vi "TirarBolaDaParede.vi"(8 "Parede":T6(ring), 9 "balls":T8[](array[typedef]), 10 "Robot in":T1, 11 "IA State":T7={"our_robots"=[], "enemy_robots"=[], "balls"=[], "geometry"={"field_length"=0, "field_width"=0, "goal_width"=0, "goal_depth"=0, "center_circle_radius"=0, "defense_width"=0, "defense_depth"=0, "free_kick_from_defense_dist"=0, "penalty_spot_from_field_line_dist"=0, "penalty_line_from_spot_dist"=0, "half_moon_depth"=0, "half_moon_width"=0}, "IA Judge"={"stage"="", "command"="", "our_goalie_id"=0.0, "enemy_goalie_id"=0.0, "command enum"=enum."Halt", "Time"=enum."Azul"}, "Received Timestamp"=timestamp(0 s since 1904-01-01), "Events"={"Touch"=FALSE, "id touch"=0.0, "Ball out of \nVision"=FALSE, "Ball inside \nGoalie area"=FALSE, "Robot not responding"=FALSE, "Robots responding status"=[1.0, 1.0, 1.0, 1.0, 1.0, 1.0], "Enemy Ball \nPossession"=FALSE, "Id ini Possession"=0.0, "Ball Possesion"=FALSE, "Id Possesion"=0.0, "Ball at\nour goal side"=FALSE, "Ball at\ntouchline"=FALSE, "Ball at\nenemy goal side"=FALSE}}) -> (3 "Cluster de saída":T1)   [LabVIEW 2018]
doc: "Função que lida com o atacante quando em \"Tirar a bola da parede\"."
uses:
  Core/AI Robot.ctl
  Intel/Functions Enum.ctl
  Intel/AttackerStates.ctl
  Path Planning/RRT/PathDests.ctl
  Path Planning/RRT/PathDest.ctl
  Core/AI Ball.ctl
  Core/AI Input.ctl
  Core/Field Size.ctl
  Core/AI Judge.ctl
  Intel/Command Enum.ctl
  Util/Events/Events.ctl
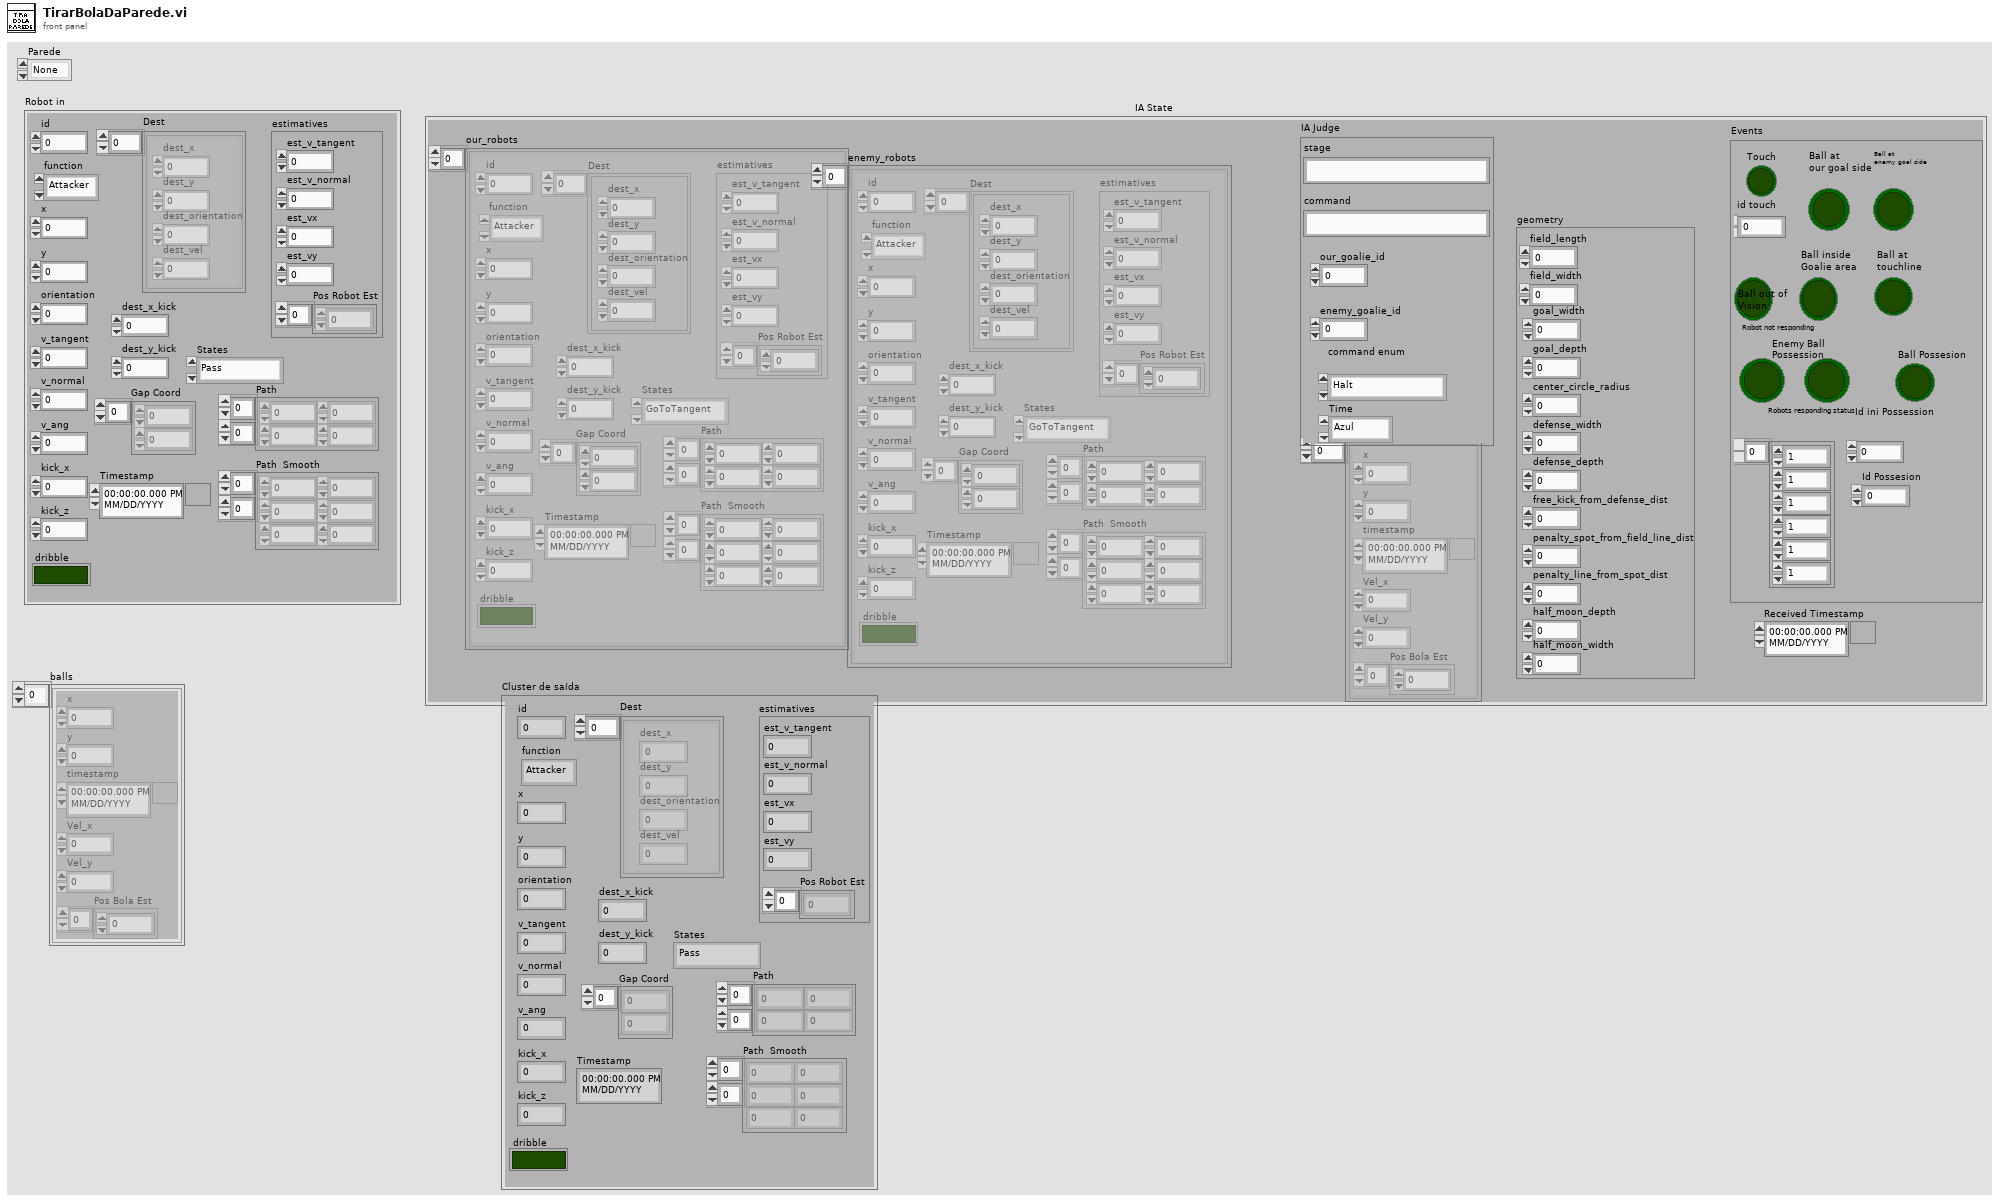
[diagram p1: front panel]
types:
  T1 = typedef "AI Robot.ctl" = cluster{"id":u32, "function":T2, "x":dbl, "y":dbl, "orientation":dbl, "v_tangent":dbl, "v_normal":dbl, "v_ang":dbl, "kick_x":dbl, "kick_z":dbl, "dribble":bool, "Timestamp":timestamp, "estimatives":cluster{"est_v_tangent":dbl, "est_v_normal":dbl, "est_vx":dbl, "est_vy":dbl, "Pos Robot Est":dbl[]}, "dest_x_kick":dbl, "dest_y_kick":dbl, "Gap Coord":dbl[], "States":T3, "Path ":dbl[][], "Path  Smooth":dbl[][], "Dest":T4}
  T2 = typedef "Functions Enum.ctl" = enum16{"Attacker", "Goalie", "Defender", "Striker", "Goto 0", "Dummy", "Kicker", "ZigZag"}
  T3 = typedef "AttackerStates.ctl" = enum16{"Pass", "GoToTangent", "BallGetting", "GoToKick", "Rotate anti-clockwise", "Rotate Clockwise", ""}
  T4 = typedef "PathDests.ctl" = T5[]
  T5 = typedef "PathDest.ctl" = cluster{"dest_x":dbl, "dest_y":dbl, "dest_orientation":dbl, "dest_vel":dbl}
  T6 = enum16{"None", "Frente", "Trás", "Cima", "Baixo"}
  T7 = typedef "AI Input.ctl" = cluster{"our_robots":T1[], "enemy_robots":T1[], "balls":T8[], "geometry":T9, "IA Judge":T10, "Received Timestamp":timestamp, "Events":T12}
  T8 = typedef "AI Ball.ctl" = cluster{"x":dbl, "y":dbl, "timestamp":timestamp, "Vel_x":dbl, "Vel_y":dbl, "Pos Bola Est":dbl[]}
  T9 = typedef "Field Size.ctl" = cluster{"field_length":u32, "field_width":u32, "goal_width":u32, "goal_depth":u32, "center_circle_radius":u32, "defense_width":u32, "defense_depth":u32, "free_kick_from_defense_dist":u32, "penalty_spot_from_field_line_dist":u32, "penalty_line_from_spot_dist":u32, "half_moon_depth":u32, "half_moon_width":u32}
  T10 = typedef "AI Judge.ctl" = cluster{"stage":string, "command":string, "our_goalie_id":dbl, "enemy_goalie_id":dbl, "command enum":T11, "Time":enum16{"Azul", "Amarelo"}}
  T11 = typedef "Command Enum.ctl" = enum16{"Halt", "Stop", "Force Start", "PKA Normal Start", "Prepare Kickoff Ally", "PKE Normal Start", "Prepare Kickoff Enemy", "Prepare Penalty Ally", "PPA Normal Start", "Prepare Penalty Enemy", "PPE Normal Start", "Ball Placement Enemy Up", "Ball Placement Enemy Down", "Ball Placement Ally Up", "Ball Placement Ally Mid", "Ball Placement Ally Down", "Indirect Free Enemy", "Indirect Free Ally", "Timeout Enemy", "Timeout Ally", "Goal Enemy", "Goal Ally", "Normal Half Time", "Extra Time Break", "Extra Half Time", "None", "Post Game"}
  T12 = typedef "Events.ctl" = cluster{"Touch":bool, "id touch":dbl, "Ball out of \nVision":bool, "Ball inside \nGoalie area":bool, "Robot not responding":bool, "Robots responding status":dbl[], "Enemy Ball \nPossession":bool, "Id ini Possession":dbl, "Ball Possesion":bool, "Id Possesion":dbl, "Ball at\nour goal side":bool, "Ball at\ntouchline":bool, "Ball at\nenemy goal side":bool}
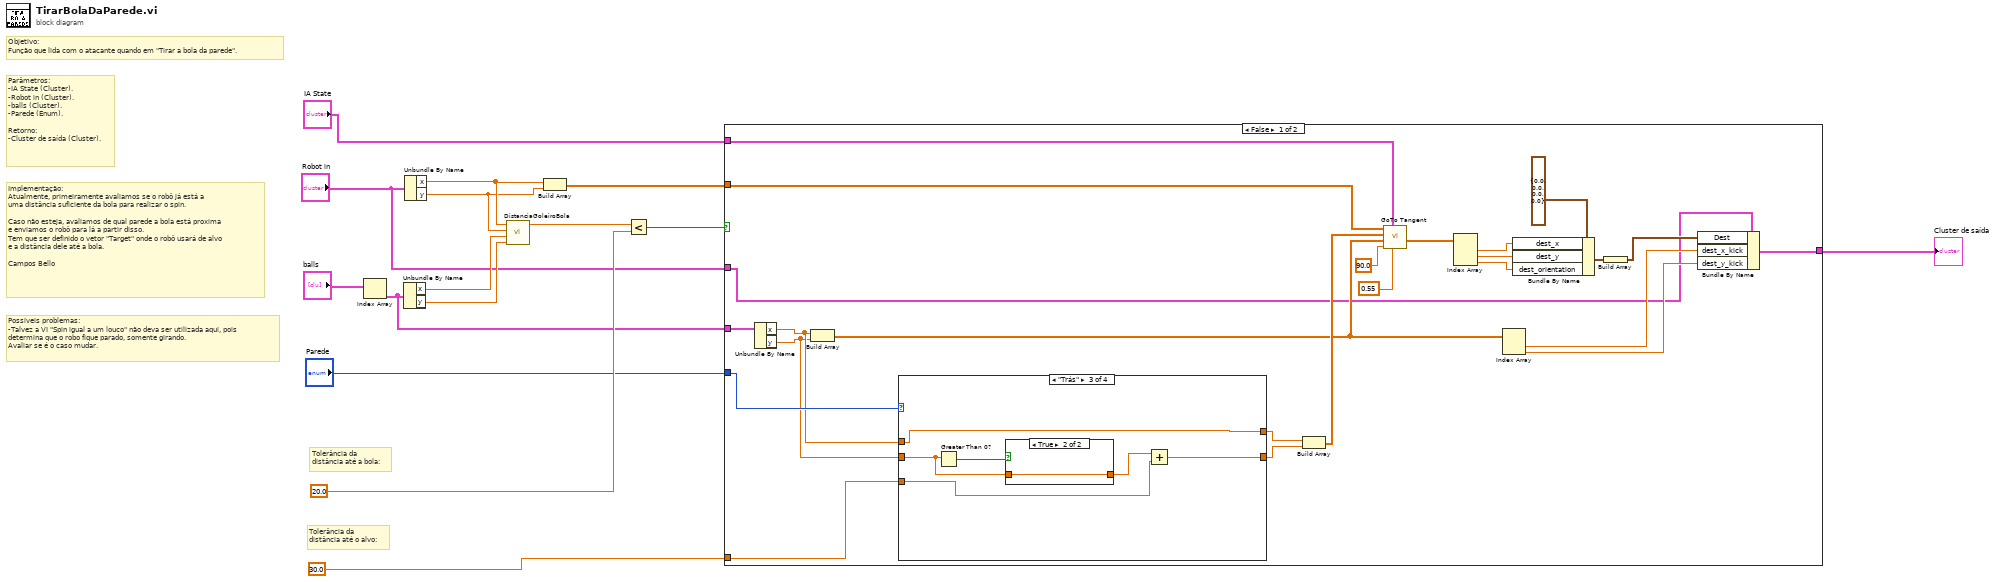
[diagram p0: block diagram]
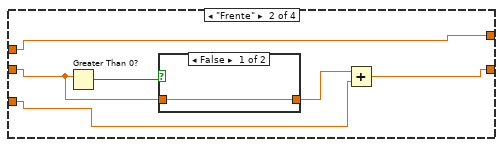
[diagram p3: hidden frame]
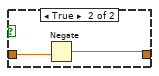
[diagram p4: hidden frame]
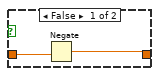
[diagram p5: hidden frame]
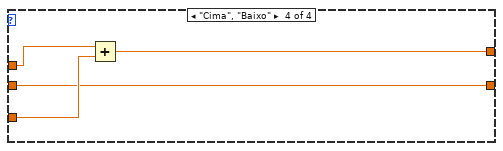
[diagram p6: hidden frame]
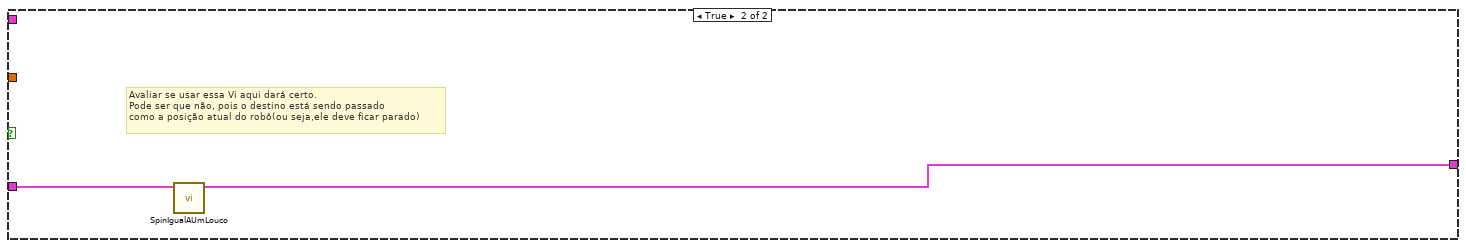
[diagram p7: hidden frame]
diagram:
  # "Possiveis problemas:\n-Talvez a VI \"Spin igual a um louco\" não deva ser utilizada aqui, pois\ndetermina que o robo fique parado, somente girando.\nAvaliar se é o caso mudar."
  # "Implementação:\nAtualmente, primeiramente avaliamos se o robô já está a\numa distância suficiente da bola para realizar o spin.\n\nCaso não esteja, avaliamos de qual parede a bola está proxima\ne enviamos o robô para lá a partir disso.\nTem que ser definido o vetor \"Target\" onde o robô usará de alvo\ne a distância dele até a bola.\n\nCampos Bello"
  # "Parâmetros:\n-IA State (Cluster).\n-Robot in (Cluster).\n-balls (Cluster).\n-Parede (Enum).\n\nRetorno:\n-Cluster de saída (Cluster)."
  # "Objetivo:\nFunção que lida com o atacante quando em \"Tirar a bola da parede\"."
  # "Tolerância da\ndistância até o alvo:"
  # "Tolerância da\ndistância até a bola:"
  n1 = Index Array(array="balls") -> (element=w8:T8)  [unwired: 1 in]
  n2 = Unbundle By Name(w8) -> ("x"=w14:dbl, "y"=w13:dbl)
  n3 = Unbundle By Name("Robot in") -> ("x"=w7:dbl, "y"=w6:dbl)
  n4 = call "DistanciaGoleiroBola.vi"("Y bola"=w13, "X bola"=w14, "Y goleiro"=w6, "X goleiro"=w7) -> ("Distância"=w12:dbl)  [unwired: 7 in]
  n5 = Build Array(w7, w6) -> (w5:dbl[])
  n6 = Less?(x=w12, y=20.0) -> (x < y?=w10:bool)
  n7 = case shown="False" w10 {
    tunnel: "Robot in" -> [w17 w65]
    tunnel: [w16 w64] -> w1
    tunnel: w8 -> [w39 _]
    tunnel: w5 -> [w38 _]
    tunnel: "IA State" -> [w37 _]
    tunnel: "Parede" -> [w34 _]
    tunnel: 30.0 -> [w31 _]
    frame False {
      n8 = Unbundle By Name(w39) -> ("x"=w33:dbl, "y"=w32:dbl)
      n9 = Build Array(w33, w32) -> (w21:dbl[])
      n10 = case shown="\"Trás\"" w34 {
        tunnel: w33 -> [w41 w44 w52 w63]
        tunnel: w32 -> [w40 w45 w55 w61]
        tunnel: w31 -> [_ w42 w53 w62]
        tunnel: [w40 w43 w51 w61] -> w29
        tunnel: [w41 w44 w52 w60] -> w30
        frame "None", Default {
        }
        frame "Frente" {
          n11 = Greater Than 0?(x=w45) -> (x > 0?=w47:bool)
          n12 = case shown="False" w47 {
            tunnel: w45 -> [w48 w50]
            tunnel: [w48 w49] -> w46
            frame False {
            }
            frame True {
              n13 = Negate(x=w50) -> (-x=w49:dbl)
            }
          }
          n14 = Add(x=w46, y=w42) -> (x+y=w43:dbl)
        }
        frame "Trás" {
          n15 = Greater Than 0?(x=w55) -> (x > 0?=w56:bool)
          n16 = case shown="True" w56 {
            tunnel: w55 -> [w58 w59]
            tunnel: [w57 w59] -> w54
            frame False {
              n17 = Negate(x=w58) -> (-x=w57:dbl)
            }
            frame True {
            }
          }
          n18 = Add(x=w54, y=w53) -> (x+y=w51:dbl)
        }
        frame "Cima", "Baixo" {
          n19 = Add(x=w63, y=w62) -> (x+y=w60:dbl)
        }
      }
      n20 = Build Array(w30, w29) -> (w28:dbl[])
      n21 = call "GoTo Tangent.vi"("Cone de chute"=0.55, "IA State Input in"=w37, "distance between ball and robot"=90.0, "Ball"=w21, "Target"=w28, "R"=w38) -> ("Destination"=w27:dbl[])  [unwired: 4 in, 1 out]
      n22 = Index Array(array=w27) -> (element #1=w24:dbl, element #2=w23:dbl, element #3=w22:dbl)  [unwired: 3 in]
      n23 = Index Array(array=w21) -> (element #1=w19:dbl, element #2=w18:dbl)  [unwired: 2 in]
      n24 = Bundle By Name(cluster=T5 {"dest_x"=0.0, "dest_y"=0.0, "dest_orientation"=0.0, "dest_vel"=0.0} ("element"), "dest_x"=w24, "dest_y"=w23, "dest_orientation"=w22) -> (w25:T5)
      n25 = Build Array(w25) -> (w20:T5[])
      n26 = Bundle By Name(cluster=w17, "Dest"=w20, "dest_x_kick"=w19, "dest_y_kick"=w18) -> (w16:T1)
    }
    frame True {
      # "Avaliar se usar essa Vi aqui dará certo.\nPode ser que não, pois o destino está sendo passado\ncomo a posição atual do robô(ou seja,ele deve ficar parado)"
      n27 = call "SpinIgualAUmLouco.vi"("Robot in"=w65) -> ("Cluster de saída"=w64:T1)  [unwired: 10 in]
    }
  }
  "Cluster de saída" <- w1
